vi "Handle Drag Over.vi"(8 "error in (no error)":errorcluster, 10 "Coords":T2, 11 "Test Executive View in":refnum<class "Test Executive View.lvclass">) -> (0 "error out":errorcluster, 2 "Discard?":bool, 3 "Test Executive View out":refnum<class "Test Executive View.lvclass">)   [LabVIEW 2017, in "Test Executive View.lvclass"]
uses:
  <vilib>/gpm_packages/@cs/Test-executive-builder/Example/Application/Test Executive View/Test Executive View/Test Executive View.lvclass
  C:/Program Files/National Instruments/LabVIEW 2017/vi.lib/gpm_packages/@cs/Test-executive-builder/Source/Test Executive Builder View/Test Executive Builder View/Test Executive Builder View.lvclass
  <vilib>/Utility/miscctls.llb/LVPoint32TypeDef.ctl
  <vilib>/gpm_packages/@cs/Test-executive-builder/Source/Application Dependencies/Relative Click Location.ctl
  <vilib>/gpm_packages/@cs/Test-executive-builder/Source/Test Executive Builder View/Test Executive Builder View/Test Executive Builder View.lvclass/Test Executive Builder View.ctl
  <vilib>/gpm_packages/@cs/Test-executive-builder/Source/Test Executive Builder View/Tree Click Interpreter/Tree Click Interpreter.lvclass
  <vilib>/gpm_packages/@cs/Test-executive-builder/Source/Test Executive Builder View/Test Executive Builder View/Test Executive Builder View.lvclass
panel:
  out "Relative Click Location":T1
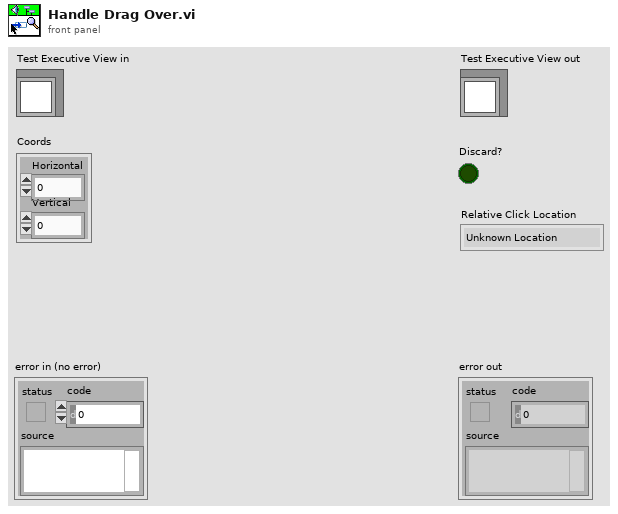
[diagram p1: front panel]
types:
  T1 = typedef "Relative Click Location.ctl" = enum16{"Unknown Location", "Below Element", "On Element", "Above Element"}
  T2 = typedef "LVPoint32TypeDef.ctl" = cluster{"Horizontal":i32, "Vertical":i32}
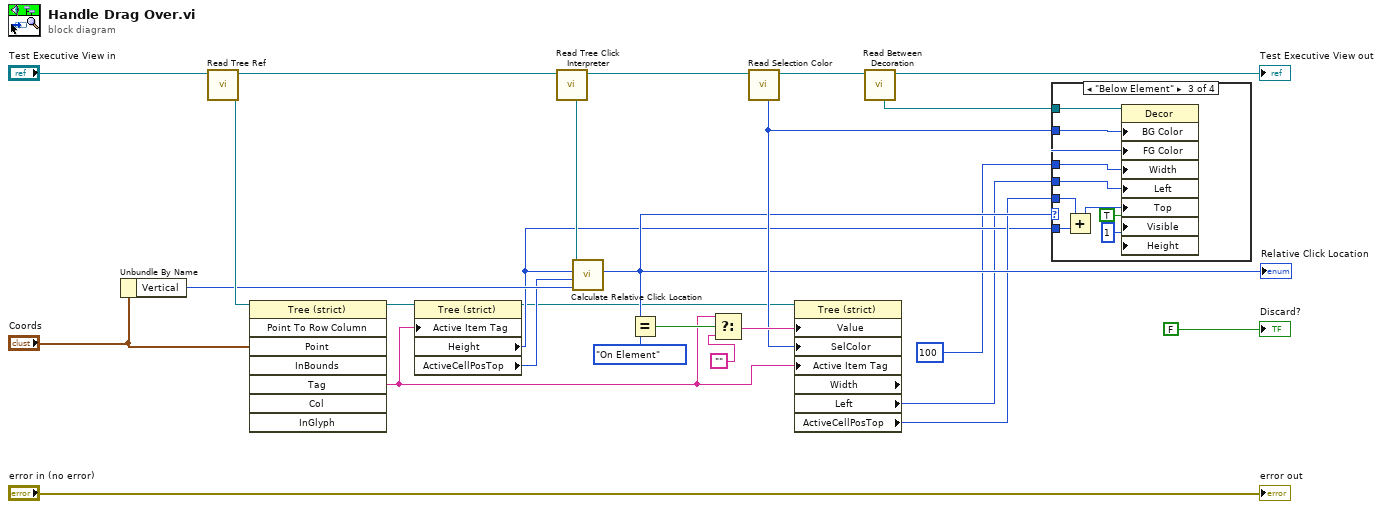
[diagram p0: block diagram]
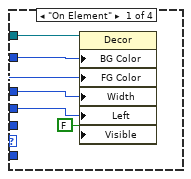
[diagram p2: hidden frame]
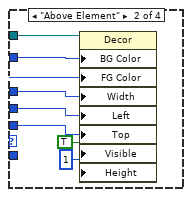
[diagram p3: hidden frame]
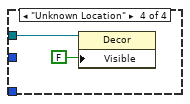
[diagram p4: hidden frame]
diagram:
  n1 = Unbundle By Name("Coords") -> ("Vertical"=w18:i32)
  n2 = call <vilib>:"Read Tree Ref.vi"("Test Executive Builder View in"="Test Executive View in") -> ("Tree Ref"=w21:refnum<vi>, "Test Executive Builder View out"=w23:refnum<class "Test Executive View.lvclass">)  [unwired: 9 in]
  n3 = invoke class="Tree (strict)" method="Point To Row Column"(reference=w21, "Point"="Coords") -> (reference out=w20:refnum<vi>, "Tag"=w3:string)  [unwired: 6 in, 6 out]
  n4 = property class="Tree (strict)"(reference=w20, "Active Item Tag"=w3) -> (reference out=w4:refnum<vi>, "Height"=w5:i32, "ActiveCellPosTop"=w17:i32)  [unwired: 1 in, 1 out]
  n5 = call <vilib>:"Read Tree Click Interpreter.vi"("Test Executive Builder View in"=w23) -> ("Test Executive Builder View out"=w12:refnum<class "Test Executive View.lvclass">, "Tree Click Interpreter"=w22:refnum<class "Tree Click Interpreter.lvclass">)  [unwired: 9 in]
  n6 = call-dynamic "Calculate Relative Click Location.vi"("Click Vertical Position"=w18, "Cell Top Position"=w17, "Cell Height"=w5, "Tree Click Interpreter in"=w22) -> ("Relative Click Location"=w7:T1)  [unwired: 6 in, 1 out]
  "Relative Click Location" <- w7
  n7 = Equal?(x=w7, y=Relative_Click_Location."On Element" ("Relative Click Location")) -> (x = y?=w15:bool)
  n8 = Select(t=w3, s=w15, f="") -> (s? t:f=w14:string)
  n9 = call <vilib>:"Read Selection Color.vi"("Test Executive Builder View in"=w12) -> ("Test Executive Builder View out"=w11:refnum<class "Test Executive View.lvclass">, "Selection Color"=w8:u32)  [unwired: 9 in]
  n10 = property class="Tree (strict)" props=["Value", "SelColor", "Active Item Tag", "Width", "Left", "ActiveCellPosTop"](reference=w4, "Value"=w14, "SelColor"=w8, "Active Item Tag"=w3) -> ("Left"=w2:i32, "ActiveCellPosTop"=w6:i32)  [unwired: 1 in, 3 out]
  n11 = call <vilib>:"Read Between Decoration.vi"("Test Executive Builder View in"=w11) -> ("Test Executive Builder View out"=→"Test Executive View out":refnum<class "Test Executive View.lvclass">, "Between Decoration"=w9:refnum<vi>)  [unwired: 9 in]
  n12 = case shown="\"Below Element\"" w7 {
    tunnel: w9 -> [w31 w38 w47 w49]
    tunnel: w8 -> [w30 w37 w46 _]
    tunnel: 100 ("Active Cell:Cell Size:Width") -> [w29 w36 w45 _]
    tunnel: w2 -> [w28 w35 w44 _]
    tunnel: w6 -> [_ w33 w41 _]
    tunnel: w5 -> [_ _ w42 _]
    frame "On Element" {
      n13 = property class="Decor"(reference=w31, "BG Color"=w30, "FG Color"=w30, "Width"=w29, "Left"=w28, "Visible"=FALSE) -> ()  [unwired: 1 in, 2 out]
    }
    frame "Above Element" {
      n14 = property class="Decor"(reference=w38, "BG Color"=w37, "FG Color"=w37, "Width"=w36, "Left"=w35, "Top"=w33, "Visible"=TRUE, "Height"=u32 1 ("Size:Height")) -> ()  [unwired: 1 in, 2 out]
    }
    frame "Below Element" {
      n15 = Add(x=w41, y=w42) -> (x+y=w40:i32)
      n16 = property class="Decor"(reference=w47, "BG Color"=w46, "FG Color"=w46, "Width"=w45, "Left"=w44, "Top"=w40, "Visible"=TRUE, "Height"=u32 1 ("Size:Height")) -> ()  [unwired: 1 in, 2 out]
    }
    frame "Unknown Location" {
      n17 = property class="Decor"(reference=w49, "Visible"=FALSE) -> ()  [unwired: 1 in, 2 out]
    }
  }
  "error out" <- "error in (no error)"
  "Discard?" <- FALSE ("Discard?")
